vi "Read Dependency list.vi"(11 "CDependencyList in":refnum<class "CDependencyList.lvclass">) -> (2 "Dependency List":T1, 3 "CDependencyList out":refnum<class "CDependencyList.lvclass">)   [LabVIEW 2020, in "DependencyInspection.lvlib" / "CDependencyList.lvclass"]
uses:
  CDependencyList.lvclass
  LabVIEWObjectInterfaces/ILabVIEWItem/ILabVIEWItem.lvclass
  DependencyList.ctl
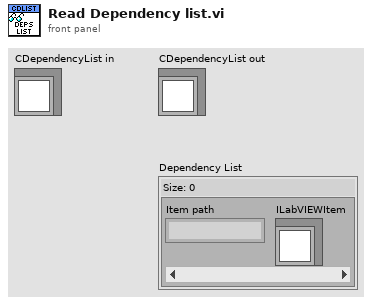
[diagram p1: front panel]
types:
  T1 = typedef "DependencyInspection.lvlib/CDependencyList.lvclass/DependencyList.ctl" = map{string, refnum<class "ILabVIEWItem.lvclass">}
  T2 = typedef "DependencyInspection.lvlib/CDependencyList.lvclass/DependencyListRef.ctl" = refnum<data-value>
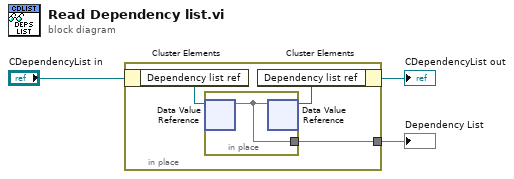
[diagram p0: block diagram]
diagram:
  n1 = in-place {
    in-place-border: [w6] -> w1
    n2 = in-place-cluster #1("CDependencyList in") -> ("Dependency list ref"=w5:T2)
    n3 = in-place {
      in-place-border: [w7] -> w6
      n4 = in-place-dvr #2(w5) -> (w7:T1)  [unwired: 1 out]
      n5 = in-place-dvr #2(w7) -> (w4:T2)  [unwired: 1 out]
    }
    n6 = in-place-cluster #1("Dependency list ref"=w4) -> (→"CDependencyList out":refnum<class "CDependencyList.lvclass">)
  }
  "Dependency List" <- w1
